vi "Read Setup.vi"(8 "error in (no error)":errorcluster, 11 "Interface in":refnum<class "Interface.lvclass">) -> (0 "error out":errorcluster, 2 "Camera Setup":T1={"Exposure Time"=1e-05, "Readout Rate"=0, "Pre-amp gain"=0, "Initial Line"=1, "Final Line"=1024, "Final Column"=1024, "Initial Cloumn"=1, "Binning"=1, "EM Gain"=2, "EM Mode"=0, "Kinetic Series Length"=1} {"Kinetic Series Length" min=1; "EM Mode" items=["Electron Multiplying", "Conventional"]; "EM Gain" min=2 max=300; "Binning" min=1 max=2; "Initial Cloumn" min=1 max=1024; "Final Column" min=1 max=1024; "Final Line" min=1 max=1024; "Initial Line" min=1 max=1024; "Pre-amp gain" items=["Gain 1", "Gain 2"]; "Readout Rate" items=["30 MHz", "20 MHz", "10 MHz", "  1 MHz"]; "Exposure Time" min=1e-05}, 3 "Interface out":refnum<class "Interface.lvclass">)   [LabVIEW 2018, in "Interface.lvclass"]
uses:
  Interface.lvclass
  Interface.lvclass/Interface.ctl
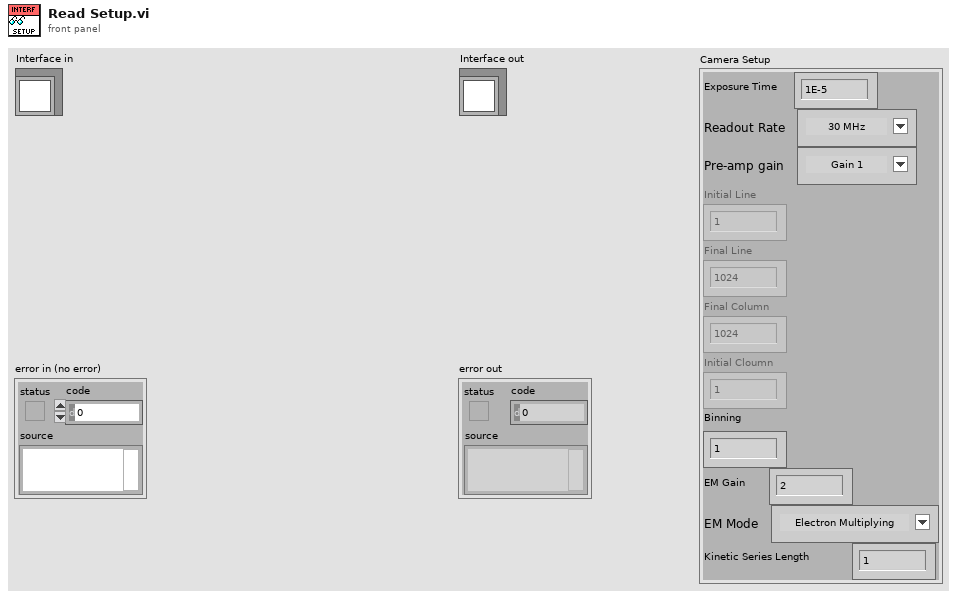
[diagram p1: front panel]
types:
  T1 = cluster{"Exposure Time":dbl, "Readout Rate":u8, "Pre-amp gain":u8, "Initial Line":u16, "Final Line":u16, "Final Column":u16, "Initial Cloumn":u16, "Binning":u8, "EM Gain":u16, "EM Mode":u8, "Kinetic Series Length":u16}
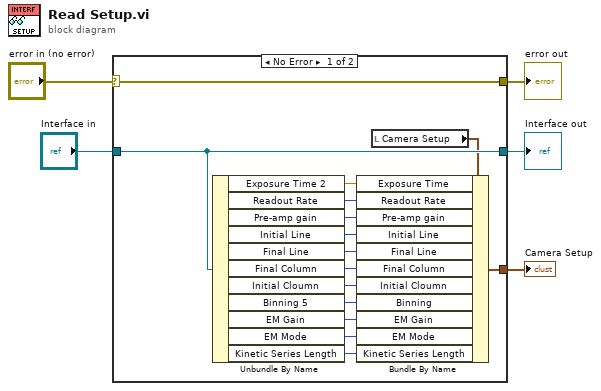
[diagram p0: block diagram]
diagram:
  n1 = case shown="No Error" "error in (no error)" {
    selector: "error in (no error)" -> [w20 w22]
    tunnel: [w20 w22] -> w4
    tunnel: [w19 w21] -> w2
    tunnel: "Interface in" -> [w19 w21]
    tunnel: [w15 _] -> w1
    frame No Error {
      n2 = Unbundle By Name(w19) -> ("Exposure Time 2"=w17:dbl, "Readout Rate"=w14:u8, "Pre-amp gain"=w13:u8, "Initial Line"=w12:u16, "Final Line"=w11:u16, "Final Column"=w10:u16, "Initial Cloumn"=w9:u16, "Binning 5"=w8:u8, "EM Gain"=w7:u32, "EM Mode"=w6:u8, "Kinetic Series Length"=w16:u16)
      n3 = local read "Camera Setup"() -> (w18:T1)
      n4 = Bundle By Name(cluster=w18, "Exposure Time"=w17, "Readout Rate"=w14, "Pre-amp gain"=w13, "Initial Line"=w12, "Final Line"=w11, "Final Column"=w10, "Initial Cloumn"=w9, "Binning"=w8, "EM Gain"=w7, "EM Mode"=w6, "Kinetic Series Length"=w16) -> (w15:T1)
    }
    frame Error {
    }
  }
  "error out" <- w4
  "Interface out" <- w2
  "Camera Setup" <- w1
